vi "MRU_GetMRULIst.vi"(8 "error in (no error)":errorcluster, 11 "reference in":refnum<class "MRU.lvclass">) -> (0 "error out":errorcluster, 3 "reference out":refnum<class "MRU.lvclass">)   [LabVIEW 2014, in "MRU.lvclass"]
doc: "Populates the ComboBox with the values in the MRU list. Uses the cached ComboBox reference passed into the constructor."
uses:
  MRU.lvclass
  <vilib>/Utility/config.llb/Read Key (String).vi
  <vilib>/Utility/config.llb/NI_LVConfig.lvlib
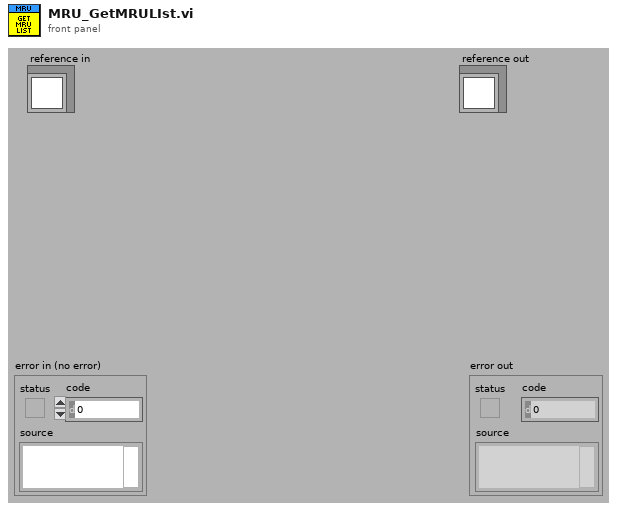
[diagram p1: front panel]
types:
  T1 = typedef "MRU.lvclass/ObjectAttributes.ctl" = cluster{"MRU INI file":path, "MRU Section Name":string, "CmbBox Refnum":refnum<vi>, "Number to remember":i32}
  T2 = typedef "NI_LVConfig.lvlib/Config Data RefNum.ctl" = refnum<k1>
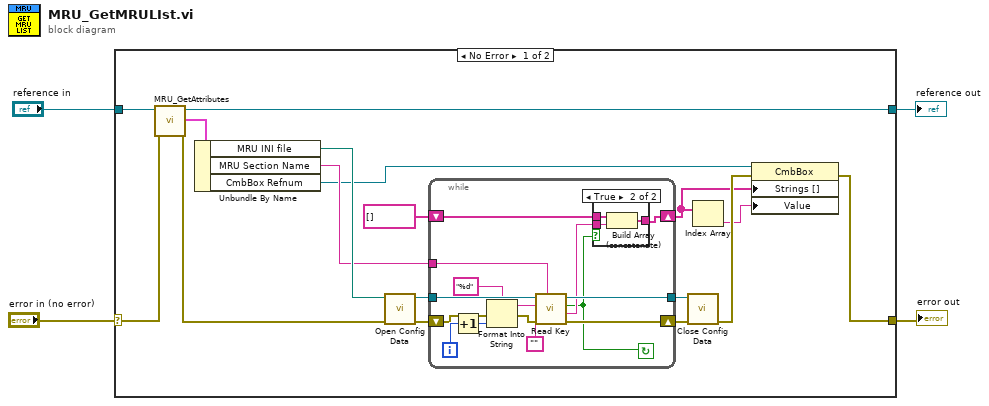
[diagram p0: block diagram]
diagram:
  n1 = case shown="No Error" "error in (no error)" {
    selector: "error in (no error)" -> [w21 w42]
    tunnel: [w8 w42] -> w3
    tunnel: [w19 w41] -> w1
    tunnel: "reference in" -> [w20 w41]
    frame No Error {
      n2 = call "MRU_GetAttributes.vi"("error in (no error)"=w21, "reference in"=w20) -> ("error out"=w9:errorcluster, "Data"=w7:T1, "reference out"=w19:refnum<class "MRU.lvclass">)  [unwired: 6 in, 1 out]
      n3 = Unbundle By Name(w7) -> ("MRU INI file"=w13:path, "MRU Section Name"=w12:string, "CmbBox Refnum"=w11:refnum<vi>)
      n4 = call <vilib>:"Open Config Data.vi"("error in (no error)"=w9, "configuration file path"=w13) -> ("error out"=w15:errorcluster, "refnum"=w17:T2)  [unwired: 7 in, 1 out]
      n5 = while {
        tunnel: w17 -> [w35]
        tunnel: [w34] -> w18
        shift-right: [w36] -> w16
        shift-left: w15 -> [w29]
        tunnel: w12 -> [w33]
        shift-right: [w24] -> w6
        shift-left: string[] [] -> [w25]
        i -> [w31]
        stop <- w23 continue-if-true
        n6 = Increment(x=w31) -> (x+1=w22:i32)
        n7 = Format Into String(format string="%d", error in=w29, w22) -> (resulting string=w30:string, error out=w28:errorcluster)  [unwired: 1 in]
        n8 = call-poly <vilib>:"Read Key.vi"("section"=w33, "error in (no error)"=w28, "default value"="", "key"=w30, "refnum"=w35) -> ("error out"=w36:errorcluster, "value"=w26:string, "found?"=w23:bool, "refnum out"=w34:T2)  [unwired: 1 in, 2 out]
        n9 = case shown="True" w23 {
          tunnel: w26 -> [_ w40]
          tunnel: w25 -> [w37 w39]
          tunnel: [w37 w38] -> w24
          frame False {
          }
          frame True {
            n10 = Build Array (concatenate)(w39, w40) -> (w38:string[])
          }
        }
      }
      n11 = call <vilib>:"Close Config Data.vi"("error in (no error)"=w16, "refnum"=w18) -> ("error out"=w10:errorcluster)  [unwired: 1 in, 8 out]
      n12 = Index Array(array=w6) -> (element=w5:string)  [unwired: 1 in]
      n13 = property class="CmbBox"(reference=w11, error in=w10, "Strings []"=w6, "Value"=w5) -> (error out=w8:errorcluster)  [unwired: 1 out]
    }
    frame Error {
    }
  }
  "error out" <- w3
  "reference out" <- w1
